vi "Manual.vi"(8 "error in (no error)":errorcluster, 10 "event source":refnum<user-event>, 11 "String":string) -> (0 "error out":errorcluster)   [LabVIEW 2025]
uses:
  <vilib>/Handler Framework/Handler Framework.lvlib
  <vilib>/Handler Framework/CmdQueue/Enqueue Single.vi
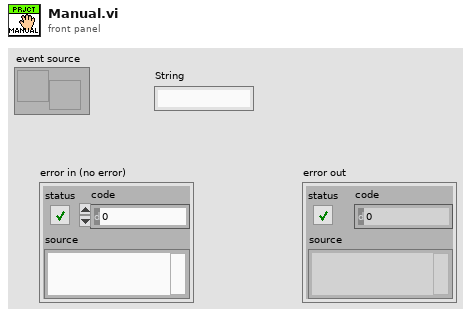
[diagram p1: front panel]
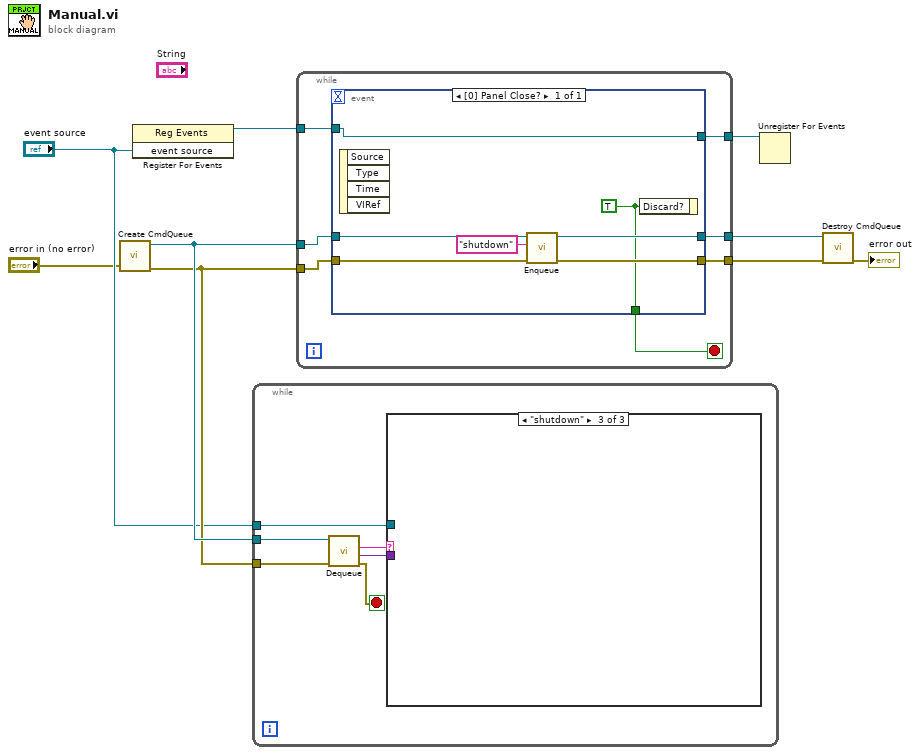
[diagram p0: block diagram]
diagram:
  n1 = call <vilib>:"Create CmdQueue.vi"("error in (no error)"="error in (no error)") -> ("error out"=w6:errorcluster, "CmdQueue out"=w7:refnum<queue>)  [unwired: 9 in]
  n2 = register-events("event source") -> (reference out=w5:refnum<event-registration>)  [unwired: 2 in, 1 out]
  n3 = while {
    tunnel: w7 -> [w15]
    tunnel: w6 -> [w11]
    tunnel: "event source" -> [w10]
    stop <- w12 stop-if-true
    n4 = call <vilib>:"Dequeue.vi"("error in (no error)"=w11, "CmdQueue in"=w15) -> ("error out"=w12:errorcluster, "value"=w13:variant, "cmd"=w14:string)  [unwired: 5 in, 2 out]
    n5 = case shown="\"shutdown\"" w14 {
      tunnel: w13 -> [_ _ _]
      tunnel: w10 -> [_ _ _]
      frame "False", Default {
      }
      frame "init" {
      }
      frame "shutdown" {
      }
    }
  }
  n6 = while {
    tunnel: w7 -> [w22]
    tunnel: [w21] -> w9
    tunnel: w6 -> [w20]
    tunnel: [w19] -> w8
    tunnel: w5 -> [w17]
    tunnel: [w16] -> w4
    stop <- w18 stop-if-true
    n7 = event shown="[0] Panel Close?" {
      selector: _ -> [_]
      dyn-events: _ -> [_]
      timeout: _ -> [_]
      tunnel: w22 -> [w29]
      tunnel: [w28] -> w21
      tunnel: w20 -> [w27]
      tunnel: [w26] -> w19
      tunnel: [w24] -> w18
      tunnel: w17 -> [w23]
      tunnel: [w23] -> w16
      event Panel Close? {
        w24 = TRUE ("Discard?")
        n8 = event-data() -> ()  [unwired: 1 in, 4 out]
        n9 = call-poly <vilib>:"Enqueue.vi"("error in (no error)"=w27, "Command"="shutdown", "CmdQueue in"=w29) -> ("error out"=w26:errorcluster, "CmdQueue out"=w28:refnum<queue>)  [unwired: 7 in]
        n10 = event-data("Discard?"=w24) -> ()  [unwired: 1 in, 1 out]
      }
    }
  }
  n11 = Unregister For Events(event registration refnum=w4) -> ()  [unwired: 1 in, 1 out]
  n12 = call <vilib>:"Destroy CmdQueue.vi"("error in (no error)"=w8, "CmdQueue in"=w9) -> ("error out"=→"error out":errorcluster)  [unwired: 9 in]
